vi "Teleop.vi"(10 "Match Info":T1={"Autonomous Elapsed Seconds"=0.0, "TeleOp Elapsed Seconds"=0.0, "Disabled Elapsed Seconds"=0.0, "Visited Autonomous"=FALSE, "Visited TeleOp"=FALSE, "Visited Disabled"=FALSE, "Autonomous Settings"={"Autonomous Style"=enum."Independent", "VI Refnum"=refnum}}, 11 "Call Context":T2) -> ()   [LabVIEW 2020]
doc: "This VI is called for each TeleOp packet received from the DS where the robot is not disabled. It is often used to read from the joysticks and update I/O or to update setpoints for timed control loops. It should complete and return within 20 milliseconds or it may miss DS packets."
uses:
  <vilib>/Rock Robotics/WPI/DriverStation/WPI_DriverStationDerivedRobotMode.ctl
  <vilib>/Rock Robotics/WPI/DriverStation/WPI_DriverStationMatch Info.ctl
  <vilib>/Rock Robotics/WPI/Utilities/WPI_GetSetVariantRefNum.vi
  Global Variable/Axes_N_Buttons.vi
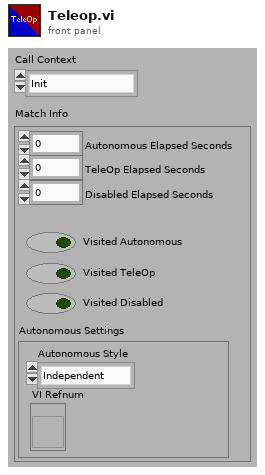
[diagram p1: front panel]
types:
  T1 = typedef "WPI_DriverStationMatch Info.ctl" = cluster{"Autonomous Elapsed Seconds":dbl, "TeleOp Elapsed Seconds":dbl, "Disabled Elapsed Seconds":dbl, "Visited Autonomous":bool, "Visited TeleOp":bool, "Visited Disabled":bool, "Autonomous Settings":cluster{"Autonomous Style":enum16{"Iterative", "Independent"}, "VI Refnum":refnum<vi>}}
  T2 = typedef "WPI_DriverStationDerivedRobotMode.ctl" = enum16{"Init", "Execute", "Stop"}
  T3 = typedef "WPI_JoystickDevRef.ctl" = cluster{"Device":T4}
  T4 = typedef "WPI_JoystickDeviceEnum.ctl" = enum16{"USB 0", "USB 1", "USB 2", "USB 3", "USB 4", "USB 5"}
  T5 = typedef "Button Cluster.ctl" = cluster{"Buttons[0]":bool, "Buttons[1]":bool, "Buttons[2]":bool, "Buttons[3]":bool, "Buttons[4]":bool, "Buttons[5]":bool, "Buttons[6]":bool, "Buttons[7]":bool, "Buttons[8]":bool, "Buttons[9]":bool}
  T6 = typedef "Axes Cluster.ctl" = cluster{"Axes[0]":dbl, "Axes[1]":dbl, "Axes[2]":dbl, "Axes[3]":dbl, "Axes[4]":dbl, "Axes[5]":dbl, "Axes[6]":dbl, "Axes[7]":dbl, "Axes[8]":dbl}
  T7 = typedef "D-Pad.ctl" = cluster{"Top":bool, "Bottom":bool, "None":bool, "Right":bool, "Left":bool}
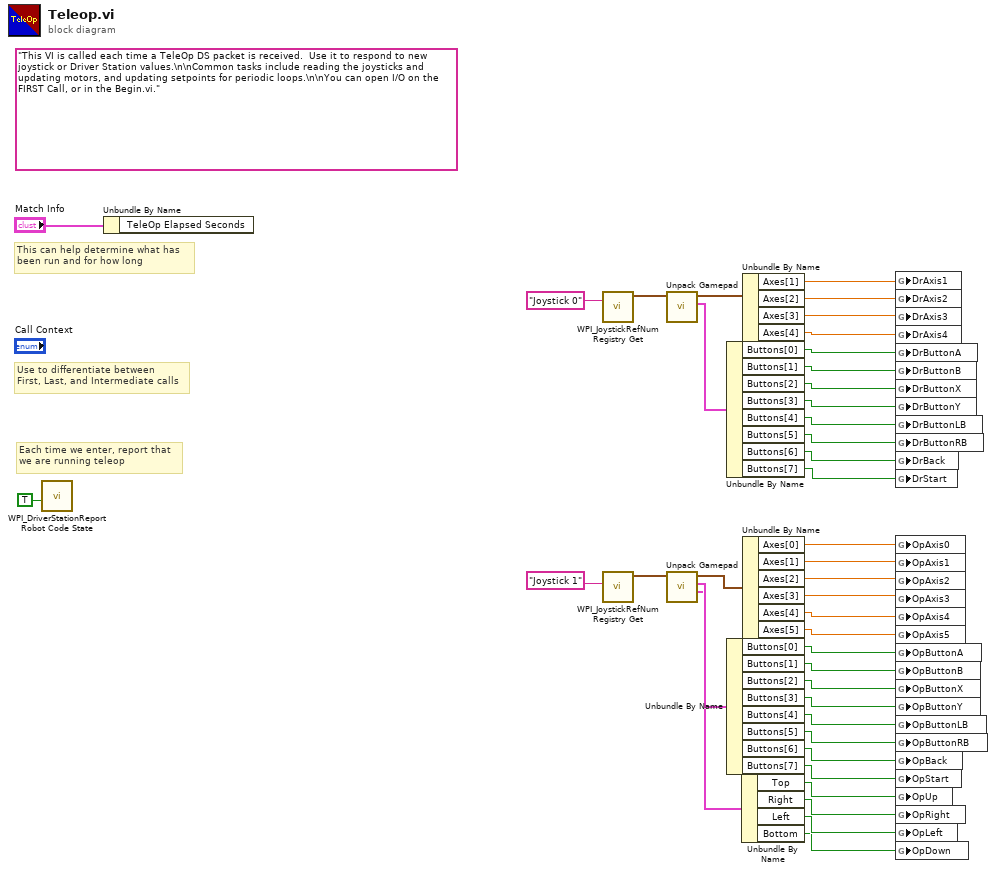
[diagram p0: block diagram]
diagram:
  (unwired) "This VI is called each time a TeleOp DS packet is received.  Use it to respond to new joystick or Driver Station values.\n\nCommon tasks include reading the joysticks and updating motors, and updating setpoints for periodic loops.\n\nYou can open I/O on the FIRST Call, or in the Begin.vi."
  # "Each time we enter, report that\nwe are running teleop"
  # "Use to differentiate between\nFirst, Last, and Intermediate calls"
  # "This can help determine what has\nbeen run and for how long"
  n1 = call <vilib>:"WPI_DriverStationReport Robot Code State.vi"("TeleOp"=TRUE ("Autonomous")) -> ()  [unwired: 10 in, 1 out]
  n2 = Unbundle By Name("Match Info") -> ()  [unwired: 1 out]
  n3 = call <vilib>:"WPI_JoystickRefNum Registry Get.vi"("refnum name"="Joystick 0") -> ("JoystickDevRef"=w36:T3)  [unwired: 1 in, 9 out]
  n4 = call <vilib>:"WPI_JoystickRefNum Registry Get.vi"("refnum name"="Joystick 1") -> ("JoystickDevRef"=w37:T3)  [unwired: 1 in, 9 out]
  n5 = call "Unpack Gamepad.vi"("JoystickDevRef"=w36) -> ("Button Cluster"=w34:T5, "Axes"=w35:T6)  [unwired: 8 in, 1 out]
  n6 = call "Unpack Gamepad.vi"("JoystickDevRef"=w37) -> ("D-Pad"=w32:T7, "Button Cluster"=w33:T5, "Axes"=w31:T6)  [unwired: 8 in]
  n7 = Unbundle By Name(w34) -> ("Buttons[0]"=w26:bool, "Buttons[1]"=w25:bool, "Buttons[2]"=w24:bool, "Buttons[3]"=w23:bool, "Buttons[4]"=w22:bool, "Buttons[5]"=w21:bool, "Buttons[6]"=w20:bool, "Buttons[7]"=w19:bool)
  n8 = Unbundle By Name(w33) -> ("Buttons[0]"=w12:bool, "Buttons[1]"=w11:bool, "Buttons[2]"=w10:bool, "Buttons[3]"=w9:bool, "Buttons[4]"=w8:bool, "Buttons[5]"=w7:bool, "Buttons[6]"=w6:bool, "Buttons[7]"=w5:bool)
  n9 = Unbundle By Name(w32) -> ("Top"=w4:bool, "Right"=w3:bool, "Left"=w2:bool, "Bottom"=w1:bool)
  n10 = Unbundle By Name(w35) -> ("Axes[1]"=w30:dbl, "Axes[2]"=w29:dbl, "Axes[3]"=w28:dbl, "Axes[4]"=w27:dbl)
  n11 = Unbundle By Name(w31) -> ("Axes[0]"=w18:dbl, "Axes[1]"=w17:dbl, "Axes[2]"=w16:dbl, "Axes[3]"=w15:dbl, "Axes[4]"=w14:dbl, "Axes[5]"=w13:dbl)
  n12 = global write "Axes_N_Buttons.vi" "DrAxis1"(w30) -> ()
  n13 = global write "Axes_N_Buttons.vi" "DrAxis2"(w29) -> ()
  n14 = global write "Axes_N_Buttons.vi" "DrAxis3"(w28) -> ()
  n15 = global write "Axes_N_Buttons.vi" "DrAxis4"(w27) -> ()
  n16 = global write "Axes_N_Buttons.vi" "DrButtonA"(w26) -> ()
  n17 = global write "Axes_N_Buttons.vi" "DrButtonB"(w25) -> ()
  n18 = global write "Axes_N_Buttons.vi" "DrButtonX"(w24) -> ()
  n19 = global write "Axes_N_Buttons.vi" "DrButtonY"(w23) -> ()
  n20 = global write "Axes_N_Buttons.vi" "DrButtonLB"(w22) -> ()
  n21 = global write "Axes_N_Buttons.vi" "DrButtonRB"(w21) -> ()
  n22 = global write "Axes_N_Buttons.vi" "DrBack"(w20) -> ()
  n23 = global write "Axes_N_Buttons.vi" "DrStart"(w19) -> ()
  n24 = global write "Axes_N_Buttons.vi" "OpAxis0"(w18) -> ()
  n25 = global write "Axes_N_Buttons.vi" "OpAxis1"(w17) -> ()
  n26 = global write "Axes_N_Buttons.vi" "OpAxis2"(w16) -> ()
  n27 = global write "Axes_N_Buttons.vi" "OpAxis3"(w15) -> ()
  n28 = global write "Axes_N_Buttons.vi" "OpAxis4"(w14) -> ()
  n29 = global write "Axes_N_Buttons.vi" "OpAxis5"(w13) -> ()
  n30 = global write "Axes_N_Buttons.vi" "OpButtonA"(w12) -> ()
  n31 = global write "Axes_N_Buttons.vi" "OpButtonB"(w11) -> ()
  n32 = global write "Axes_N_Buttons.vi" "OpButtonX"(w10) -> ()
  n33 = global write "Axes_N_Buttons.vi" "OpButtonY"(w9) -> ()
  n34 = global write "Axes_N_Buttons.vi" "OpButtonLB"(w8) -> ()
  n35 = global write "Axes_N_Buttons.vi" "OpButtonRB"(w7) -> ()
  n36 = global write "Axes_N_Buttons.vi" "OpBack"(w6) -> ()
  n37 = global write "Axes_N_Buttons.vi" "OpStart"(w5) -> ()
  n38 = global write "Axes_N_Buttons.vi" "OpUp"(w4) -> ()
  n39 = global write "Axes_N_Buttons.vi" "OpRight"(w3) -> ()
  n40 = global write "Axes_N_Buttons.vi" "OpLeft"(w2) -> ()
  n41 = global write "Axes_N_Buttons.vi" "OpDown"(w1) -> ()
